vi "Pressure Sensor-DM.vi"(2 "NXT":T2={"Hardware"="NXT", "Flattened String"=""}, 3 "Input Port":T1 items=["Port 1", "Port 2", "Port 3", "Port 4"]) -> (1 "Pressure (psi)":cluster{u16}, 4 "NXT dup":T2={"Hardware"="NXT", "Flattened String"=""} caption="NXT")   [LabVIEW 2010]
uses:
  <vilib>/NXT/Subs/LVHSConnector.ctl
  <vilib>/NXT/Block Support/NXT_InputPort.ctl
  <vilib>/NXT/Dual Mode Library/Sensors/Light_On.vi
panel:
  # "mindsensors.com\nCopyright (c) 2009 by mindsensors.com\nEmail: info (<at>) mindsensors (<dot>) com\n\nThis program is free software. You can redistribute it and/or modify\nit under the terms of the GNU General Public License as published by\nthe Free Software Foundation; version 3 of the License.\nRead the license at: http://www.gnu.org/licenses/gpl.txt"
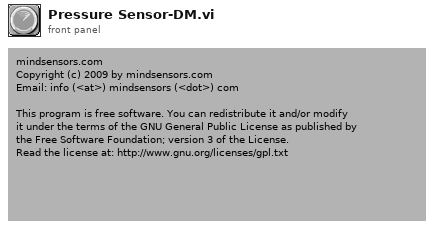
[diagram p1: front panel]
types:
  T1 = typedef "NXT_InputPort.ctl" = u8
  T2 = typedef "LVHSConnector.ctl" = cluster{"Hardware":string, "Flattened String":string}
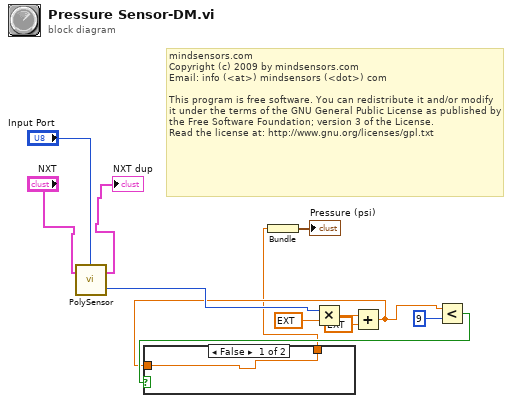
[diagram p0: block diagram]
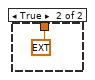
[diagram p2: hidden frame]
diagram:
  # "mindsensors.com\nCopyright (c) 2009 by mindsensors.com\nEmail: info (<at>) mindsensors (<dot>) com\n\nThis program is free software. You can redistribute it and/or modify\nit under the terms of the GNU General Public License as published by\nthe Free Software Foundation; version 3 of the License.\nRead the license at: http://www.gnu.org/licenses/gpl.txt"
  n1 = call-poly <vilib>:"PolySensor.vi"("NXT"="NXT", "Port (Port 3)"="Input Port") -> ("Scaled Value"=w8:i16, "NXT"=→"NXT dup":T2)  [unwired: 1 in]
  n2 = Multiply(x=w8, y=ext 0.28) -> (x*y=w6:ext)
  n3 = Add(x=w6, y=ext 8.67) -> (x+y=w2:ext)
  n4 = Less?(x=w2, y=i16 9) -> (x < y?=w3:bool)
  n5 = case shown="False" w3 {
    tunnel: [w13 ext 0.0] -> w1
    tunnel: w2 -> [w13 _]
    frame False {
    }
    frame True {
    }
  }
  n6 = Bundle(w1) -> (→"Pressure (psi)":cluster{ext})  [unwired: 1 in]
